vi "数据查询_校准记录.vi"() -> ()   [LabVIEW 2016]
uses:
  <vilib>/Utility/miscctls.llb/LVRowAndColumnUnsignedTypeDef.ctl
  <vilib>/Utility/miscctls.llb/LVPositionTypeDef.ctl
  <vilib>/Utility/miscctls.llb/LVPointTypeDef.ctl
  <userlib>/_OpenG.lib/array/array.llb/Sort 2D Array (String)__ogtk.vi
panel:
  in  "触发查询":bool
  out "确定查询":bool
  out "显示项":string[](array[string])
  out "condition":string
  in  "数据列表选择框":string(xcontrol)
  in  "导出":bool
  in  "条件筛选":bool
  in  "数据表":T1
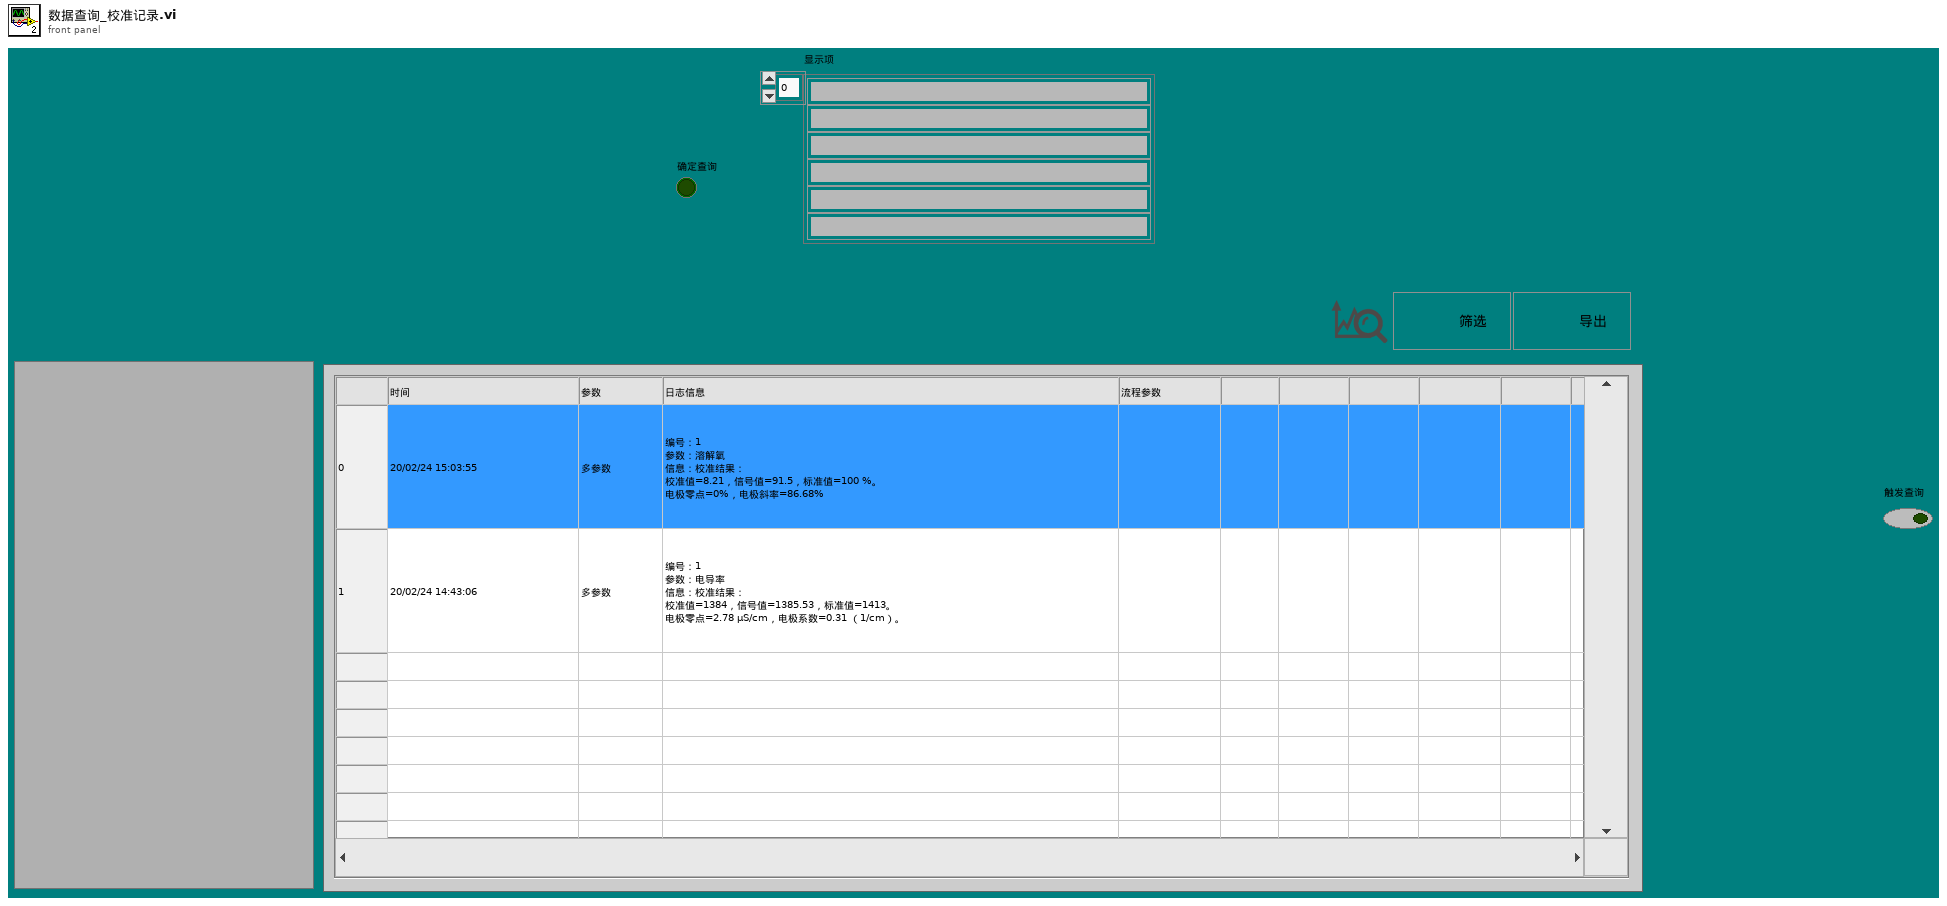
[diagram p1: front panel]
types:
  T1 = typedef "数据查询大列表框.ctl" = i32
  T2 = typedef "LVPositionTypeDef.ctl" = cluster{"Left":i32, "Top":i32}
  T3 = typedef "LVRowAndColumnUnsignedTypeDef.ctl" = cluster{"Row":u32, "Column":u32}
  T4 = typedef "LVPointTypeDef.ctl" = cluster{"Horizontal":i16, "Vertical":i16}
  T5 = enum8{"Enabled", "Disabled", "Disabled and Grayed Out"}
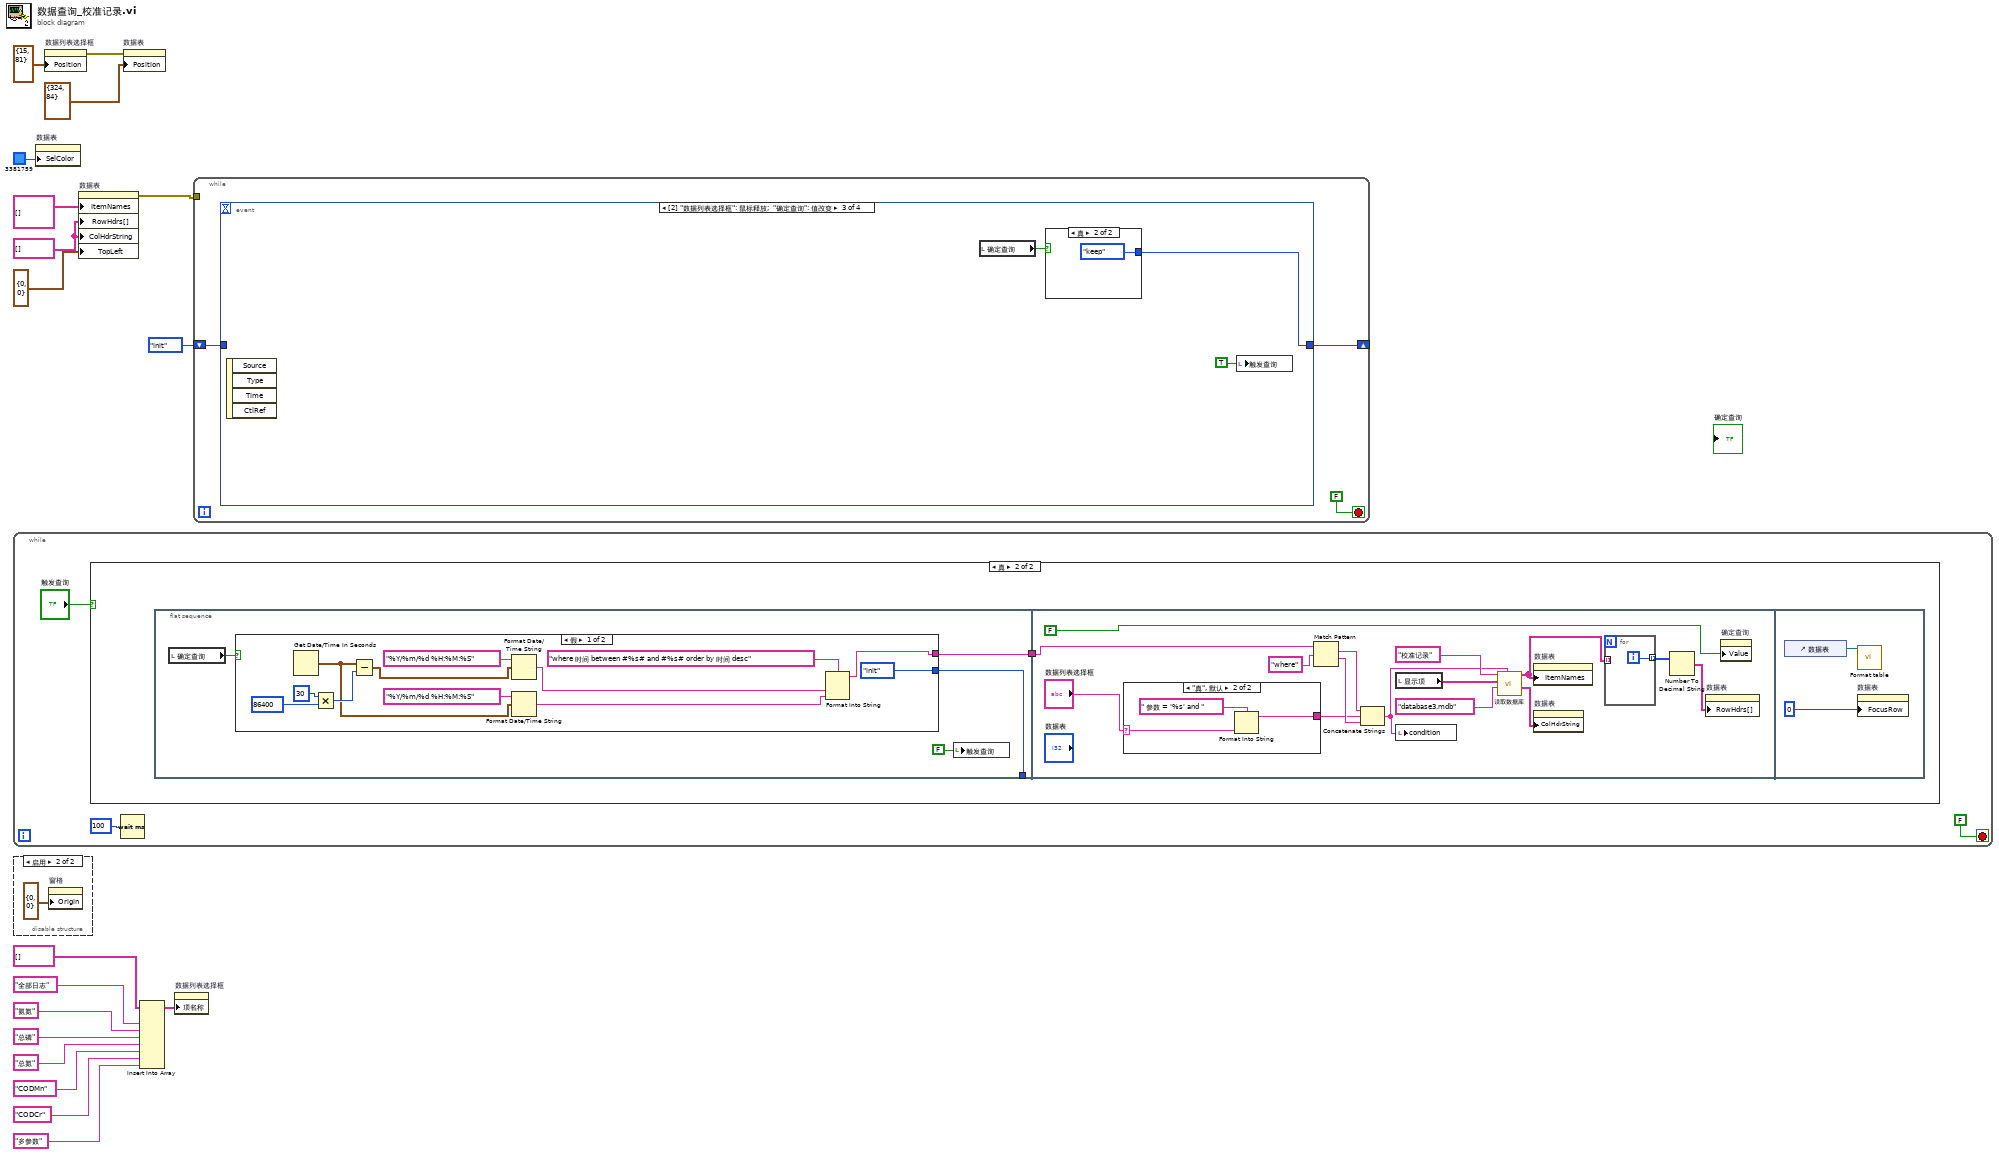
[diagram p0: block diagram]
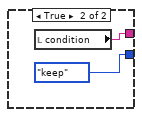
[diagram p3: hidden frame]
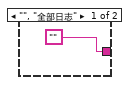
[diagram p4: hidden frame]
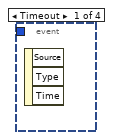
[diagram p5: hidden frame]
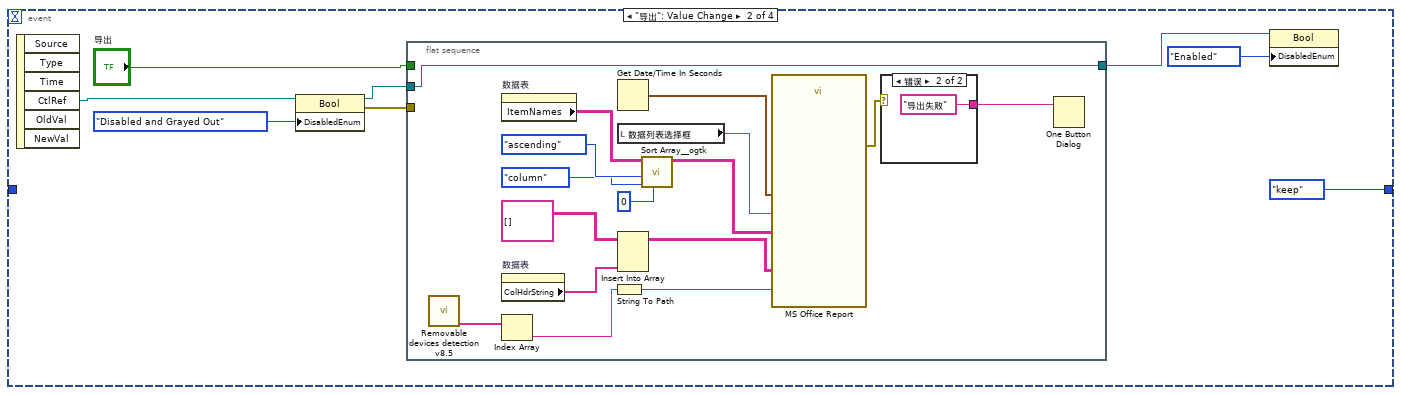
[diagram p6: hidden frame]
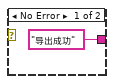
[diagram p7: hidden frame]
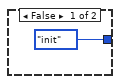
[diagram p8: hidden frame]
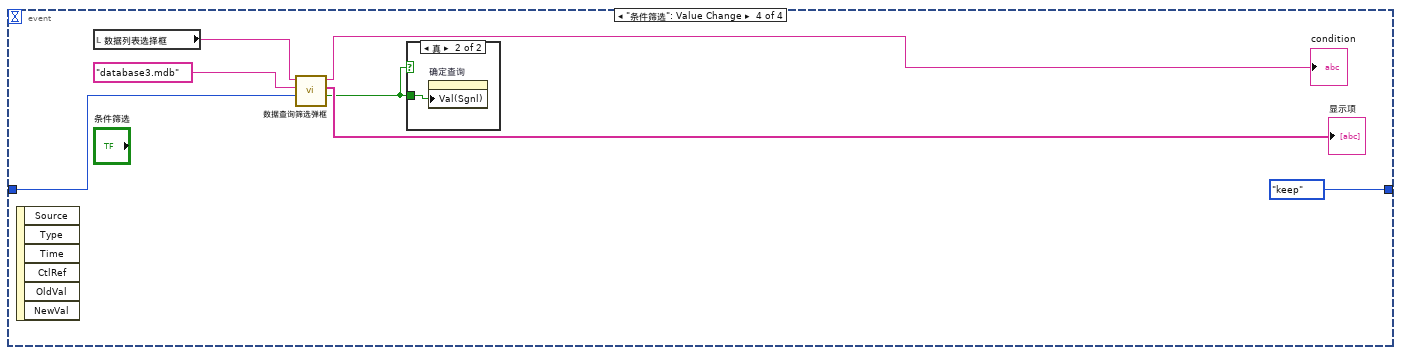
[diagram p9: hidden frame]
diagram:
  w8 = string[] [] ("行首字符串[]")
  n1 = while {
    stop <- FALSE stop-if-true
    n2 = case shown="真" "触发查询" {
      frame False {
      }
      frame True {
        n3 = flat-sequence {
          tunnel: [w25] -> w22
          tunnel: [w24] -> _
          tunnel: w22 -> [w44]
          frame #0 {
            n4 = local read "确定查询"() -> (w26:bool)
            n5 = case shown="假" w26 {
              tunnel: [w29 w39] -> w25
              tunnel: [enum16{"init", "keep"}."init" ("是否初始化") enum16{"init", "keep"}."keep" ("是否初始化")] -> w24
              frame False {
                n6 = Get Date/Time In Seconds() -> (seconds since 1Jan1904=w27:timestamp)
                n7 = Multiply(x=30, y=86400) -> (x*y=w30:i32)
                n8 = Subtract(x=w27, y=w30) -> (x-y=w35:timestamp)
                n9 = Format Date/Time String(time format string (%c)="%Y/%m/%d %H:%M:%S" ("时间格式字符串(%c)"), seconds (now)=w35) -> (date/time string=w37:string)  [unwired: 1 in]
                n10 = Format Date/Time String(time format string (%c)="%Y/%m/%d %H:%M:%S" ("时间格式字符串(%c)"), seconds (now)=w27) -> (date/time string=w38:string)  [unwired: 1 in]
                n11 = Format Into String(format string="where 时间 between #%s# and #%s# order by 时间 desc", w37, w38) -> (resulting string=w29:string)  [unwired: 2 in, 1 out]
              }
              frame True {
                n12 = local read "condition"() -> (w39:string)
              }
            }
            n13 = local write "触发查询"(FALSE ("触发查询")) -> ()
          }
          frame #1 {
            n14 = case shown="\"真\", 默认" "数据列表选择框" {
              selector: "数据列表选择框" -> [_ w58]
              tunnel: ["" w57] -> w45
              frame "", "全部日志" {
              }
              frame "真", Default {
                n15 = Format Into String(format string=" 参数 = '%s' and " ("condition"), w58) -> (resulting string=w57:string)  [unwired: 2 in, 1 out]
              }
            }
            n16 = Match Pattern(string=w44, regular expression="where") -> (match substring=w47:string, after substring=w46:string)  [unwired: 1 in, 2 out]
            n17 = Concatenate Strings(w47, w45, w46) -> (w42:string)
            n18 = local read "显示项"() -> (w43:string[])
            n19 = local write "condition"(w42) -> ()
            n20 = call "读取数据库.vi"("condition"=w42, "database"="database3.mdb", "显示项"=w43, "组合框"="校准记录" ("字符串")) -> ("columns"=w55:string[], "表格"=w50:string[][])  [unwired: 4 in, 2 out]
            n21 = property on="数据表" class="MCListbox (严格)"("ItemNames"=w50) -> ()  [unwired: 2 in, 2 out]
            n22 = property on="数据表" class="MCListbox (严格)"("ColHdrString"=w55) -> ()  [unwired: 2 in, 2 out]
            n23 = for {
              tunnel: w50 -> [_] mode=indexing
              tunnel: [w60] -> w54 mode=indexing
              i -> [w60]
            }
            n24 = Number To Decimal String(number=w54) -> (decimal integer string=w53:string[])  [unwired: 1 in]
            n25 = property on="数据表" class="MCListbox (严格)"("RowHdrs[]"=w53) -> ()  [unwired: 2 in, 2 out]
            n26 = property on="确定查询" class="Bool (严格)"("Value"=FALSE ("确定查询")) -> ()  [unwired: 2 in, 2 out]
          }
          frame #2 {
            n27 = control-ref of="数据表"() -> (w61:refnum<vi>)
            n28 = call "Format table.vi"("Table输入"=w61) -> ()  [unwired: 11 in]
            n29 = property on="数据表" class="MCListbox (严格)"("FocusRow"=0 ("选中行")) -> ()  [unwired: 2 in, 2 out]
          }
        }
      }
    }
    n30 = Wait (ms)(milliseconds to wait=u32 100 ("等待时间（毫秒）")) -> ()  [unwired: 1 out]
  }
  n31 = disable-structure shown="启用" {
    frame Disabled {
    }
    frame Enabled {
      n32 = property on="窗格" class="Pane"("Origin"=T4 {"Horizontal"=0, "Vertical"=0} ("原点")) -> ()  [unwired: 2 in, 2 out]
    }
  }
  n33 = property on="数据表" class="MCListbox (严格)"("SelColor"=u32 3381759) -> ()  [unwired: 2 in, 2 out]
  n34 = property on="数据列表选择框" class="数据列表选择框 (严格)"("Position"=T2 {"Left"=15, "Top"=81} ("位置")) -> (error out=w1:errorcluster)  [unwired: 2 in, 1 out]
  n35 = property on="数据表" class="MCListbox (严格)"("ItemNames"=string[][] [] ("项名"), "RowHdrs[]"=w8, "ColHdrString"=w8, "TopLeft"=T3 {"Row"=0, "Column"=0} ("左上可见单元格")) -> (error out=w10:errorcluster)  [unwired: 2 in, 1 out]
  n36 = property on="数据表" class="MCListbox (严格)"(error in=w1, "Position"=T2 {"Left"=324, "Top"=84} ("位置")) -> ()  [unwired: 1 in, 2 out]
  n37 = Insert Into Array(array=string[] [], new element #1="全部日志" ("新元素/子数组"), new element #2="氨氮" ("新元素/子数组"), new element #3="总磷" ("新元素/子数组"), new element #4="总氮" ("新元素/子数组"), new element #5="CODMn" ("新元素/子数组"), new element #6="CODCr" ("新元素/子数组"), new element #7="多参数" ("新元素/子数组")) -> (w6:string[])  [unwired: 1 in]
  n38 = property on="数据列表选择框" class="数据列表选择框 (严格)"("项名称"=w6) -> ()  [unwired: 2 in, 2 out]
  n39 = while {
    tunnel: w10 -> [_]
    shift-right: [w64] -> _
    shift-left: enum16{"init", "keep"}."init" ("是否初始化") -> [w65]
    stop <- FALSE stop-if-true
    n40 = event shown="[2] \"数据列表选择框\": 鼠标释放;  \"确定查询\": 值改变" {
      selector: _ -> [_ _ _ _]
      dyn-events: _ -> [_ _ _ _]
      timeout: _ -> [_ _ _ _]
      tunnel: w65 -> [_ _ _ w99]
      tunnel: [_ enum16{"init", "keep"}."keep" ("是否初始化") w94 enum16{"init", "keep"}."keep" ("是否初始化")] -> w64
      event Timeout {
        n41 = event-data() -> ()  [unwired: 1 in, 3 out]
      }
      event "导出": Value Change {
        n42 = event-data() -> ("CtlRef"=w68:refnum<vi>)  [unwired: 1 in, 5 out]
        n43 = property class="Bool"(reference=w68, "DisabledEnum"=T5."Disabled and Grayed Out" ("禁用")) -> (reference out=w72:refnum<vi>, error out=w73:errorcluster)  [unwired: 1 in]
        n44 = flat-sequence {
          tunnel: w73 -> [_]
          tunnel: [w84] -> w71
          tunnel: w72 -> [w84]
          tunnel: "导出" -> [_]
          frame #0 {
            n45 = call "Removable devices detection v8.5.vi"() -> ("Removable"=w81:string[])  [unwired: 4 out]
            n46 = property on="数据表" class="MCListbox (严格)"() -> ("ItemNames"=w75:string[][])  [unwired: 2 in, 2 out]
            n47 = property on="数据表" class="MCListbox (严格)"() -> ("ColHdrString"=w77:string[])  [unwired: 2 in, 2 out]
            n48 = Index Array(array=w81) -> (element=w80:string)  [unwired: 1 in]
            n49 = String To Path(string=w80) -> (path=w79:path)
            n50 = Get Date/Time In Seconds() -> (seconds since 1Jan1904=w90:timestamp)
            n51 = local read "数据列表选择框"() -> (w85:string)
            n52 = Insert Into Array(array=string[][] [], new element=w77) -> (w76:string[][])  [unwired: 2 in]
            n53 = call-poly <userlib>:"Sort Array__ogtk.vi"("Column/Row to Sort By"=u32 0, "Sort By in"=enum16{"row", "column"}."column", "Order"=enum16{"ascending", "descending"}."ascending", "Array in"=w75) -> ("Sorted Array out"=w89:string[][])  [unwired: 4 in, 3 out]
            n54 = call "MS Office Report"("Path to Save Report"=w79, "导出日期"=w90, "监测参数"=w85, "数据输入"=w89, "字段定义"=w76) -> ("error out"=w83:errorcluster)  [unwired: 21 in, 1 out]
            n55 = case shown="错误" w83 {
              tunnel: ["导出成功" ("消息") "导出失败" ("消息")] -> w82
              frame No Error {
              }
              frame Error {
              }
            }
            n56 = One Button Dialog(message=w82) -> ()  [unwired: 1 in, 1 out]
          }
        }
        n57 = property class="Bool"(reference=w71, "DisabledEnum"=T5."Enabled" ("禁用")) -> ()  [unwired: 1 in, 2 out]
      }
      event "数据列表选择框": Mouse Up; "确定查询": Value Change {
        n58 = event-data() -> ()  [unwired: 1 in, 4 out]
        n59 = local read "确定查询"() -> (w95:bool)
        n60 = case shown="真" w95 {
          tunnel: [enum16{"init", "keep"}."init" ("是否初始化") enum16{"init", "keep"}."keep" ("是否初始化")] -> w94
          frame False {
          }
          frame True {
          }
        }
        n61 = local write "触发查询"(TRUE ("触发查询")) -> ()
      }
      event "条件筛选": Value Change {
        n62 = event-data() -> ()  [unwired: 1 in, 6 out]
        n63 = local read "数据列表选择框"() -> (w100:string)
        n64 = call "数据查询筛选弹框.vi"("是否初始化"=w99, "database"="database3.mdb", "table"=w100) -> ("确定输出"=w102:bool, "显示项"=→"显示项":string[], "condition"=→"condition":string)  [unwired: 5 in, 1 out]
        n65 = case shown="真" w102 {
          tunnel: w102 -> [_ w105]
          frame False {
          }
          frame True {
            n66 = property on="确定查询" class="Bool (严格)"("Val(Sgnl)"=w105) -> ()  [unwired: 2 in, 2 out]
          }
        }
      }
    }
  }
